vi "DatetimeToDateTime.vi"(11 "Datetime string":string) -> (1 "Time string":string, 3 "Date string":string)   [LabVIEW 2012]
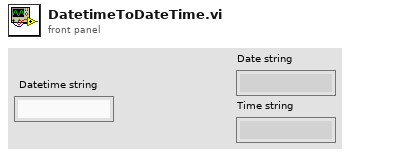
[diagram p1: front panel]
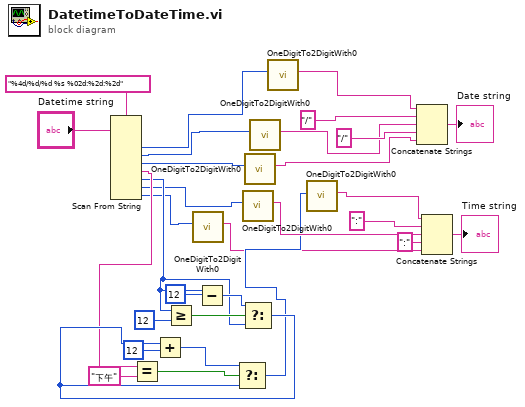
[diagram p0: block diagram]
diagram:
  n1 = Scan From String(format string="%4d/%d/%d %s %02d:%2d:%2d", input string="Datetime string") -> (output 1=w12:i32, output 2=w10:i32, output 3=w8:i32, output 4=w19:string, output 5=w18:i32, output 6=w6:i32, output 7=w2:i32)  [unwired: 9 in, 3 out]
  n2 = Equal?(x=w19, y="下午") -> (x = y?=w24:bool)
  n3 = Greater Or Equal?(x=w18, y=12) -> (x >= y?=w28:bool)
  n4 = call "OneDigitTo2DigitWith0.vi"("number"=w2) -> ("output"=w1:string)  [unwired: 10 in]
  n5 = Subtract(x=w18, y=12) -> (x-y=w26:i32)
  n6 = call "OneDigitTo2DigitWith0.vi"("number"=w6) -> ("output"=w5:string)  [unwired: 10 in]
  n7 = Select(t=w26, s=w28, f=w18) -> (s? t:f=w20:i32)
  n8 = Add(x=w20, y=12) -> (x+y=w21:i32)
  n9 = Select(t=w21, s=w24, f=w20) -> (s? t:f=w4:i32)
  n10 = call "OneDigitTo2DigitWith0.vi"("number"=w8) -> ("output"=w7:string)  [unwired: 10 in]
  n11 = call "OneDigitTo2DigitWith0.vi"("number"=w10) -> ("output"=w9:string)  [unwired: 10 in]
  n12 = call "OneDigitTo2DigitWith0.vi"("number"=w12) -> ("output"=w11:string)  [unwired: 10 in]
  n13 = call "OneDigitTo2DigitWith0.vi"("number"=w4) -> ("output"=w3:string)  [unwired: 10 in]
  n14 = Concatenate Strings(w11, "/" ("string"), w9, "/" ("string"), w7) -> (→"Date string":string)
  n15 = Concatenate Strings(w3, ":" ("string"), w5, ":" ("string"), w1) -> (→"Time string":string)
